vi "DM65-Esercitazione-1v2.vi"() -> ()   [LabVIEW 2020]
uses:
  C:/TwinCAT/AdsApi/.NET/v4.0.30319/TwinCAT.Ads.dll
  TwinCAT/AdsApi/.NET/v4.0.30319/TwinCAT.Ads.dll
panel:
  out "FUP":bool
  out "MDN":bool
  out "FDN":bool
  out "MUP":bool
  out "box":bool
  in  "fotocellula":bool
  in  "sensore":bool
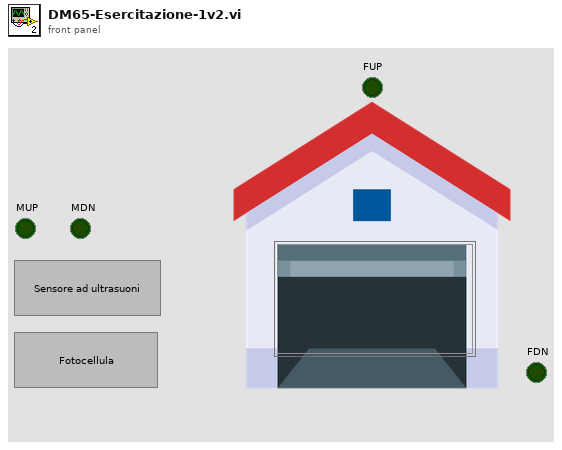
[diagram p1: front panel]
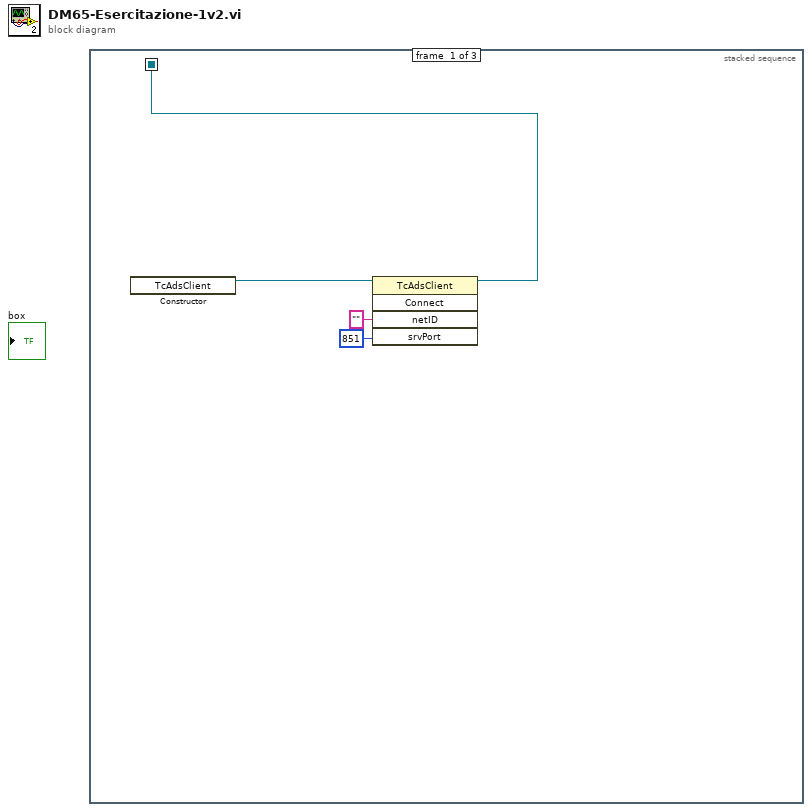
[diagram p0: block diagram]
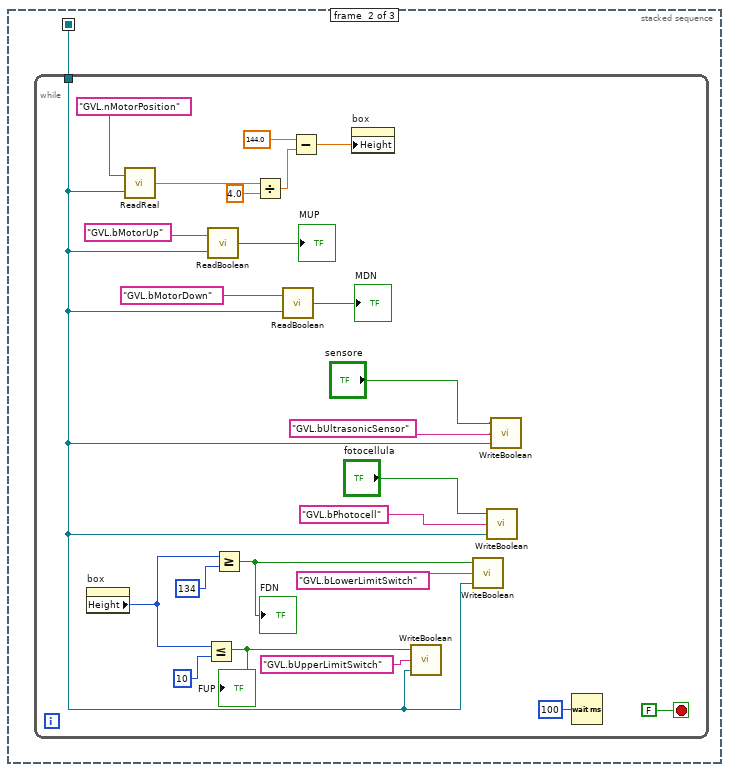
[diagram p2: hidden frame]
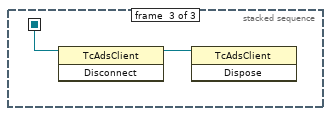
[diagram p3: hidden frame]
diagram:
  n1 = stacked-sequence {
    seq-local: [w1 _ _] -> [_ w5 w30]
    frame #0 {
      n2 = constructor class="TcAdsClient"() -> (reference out=w4:refnum<k24>)  [unwired: 3 in, 2 out]
      n3 = invoke class="TcAdsClient" method="Connect"(reference=w4, "netID"="", "srvPort"=851) -> (reference out=w1:refnum<k24>)  [unwired: 2 in, 4 out]
    }
    frame #1 {
      n4 = while {
        tunnel: w5 -> [w6]
        stop <- FALSE stop-if-true
        n5 = property on="box" class="Bool (strict)"() -> ("Height"=w15:u32)  [unwired: 2 in, 2 out]
        n6 = call "ReadReal.vi"("reference"=w6, "symbolPath"="GVL.nMotorPosition" ("name")) -> ("output"=w8:dbl)
        n7 = Less Or Equal?(x=w15, y=u32 10) -> (x <= y?=w13:bool)
        "FUP" <- w13
        n8 = call "ReadBoolean.vi"("reference"=w6, "symbolPath"="GVL.bMotorUp" ("name")) -> ("output"=→"MUP":bool)
        n9 = Greater Or Equal?(x=w15, y=u32 134) -> (x >= y?=w17:bool)
        "FDN" <- w17
        n10 = Divide(x=w8, y=4.0) -> (x/y=w23:dbl)
        n11 = call "ReadBoolean.vi"("reference"=w6, "symbolPath"="GVL.bMotorDown" ("name")) -> ("output"=→"MDN":bool)
        n12 = Subtract(x=144.0, y=w23) -> (x-y=w24:dbl)
        n13 = property on="box" class="Bool (strict)"("Height"=w24) -> ()  [unwired: 2 in, 2 out]
        n14 = call "WriteBoolean.vi"("reference"=w6, "symbolPath"="GVL.bUpperLimitSwitch", "value"=w13) -> ()
        n15 = call "WriteBoolean.vi"("reference"=w6, "symbolPath"="GVL.bLowerLimitSwitch", "value"=w17) -> ()
        n16 = call "WriteBoolean.vi"("reference"=w6, "symbolPath"="GVL.bPhotocell", "value"="fotocellula") -> ()
        n17 = call "WriteBoolean.vi"("reference"=w6, "symbolPath"="GVL.bUltrasonicSensor", "value"="sensore") -> ()
        n18 = Wait (ms)(milliseconds to wait=u32 100) -> ()  [unwired: 1 out]
      }
    }
    frame #2 {
      n19 = invoke class="TcAdsClient" method="Disconnect"(reference=w30) -> (reference out=w31:refnum<k24>)  [unwired: 2 in, 2 out]
      n20 = invoke class="TcAdsClient" method="Dispose"(reference=w31) -> ()  [unwired: 2 in, 3 out]
    }
  }
